vi "FW shifter.vi"() -> (0 "Cluster":T1)   [LabVIEW 2010, in "lib1299.lvlib"]
doc: "This is the constant for the variables used in the shift register of the firmware loader VI."
uses:
  lib1299.lvlib
  Controls/FW State.ctl
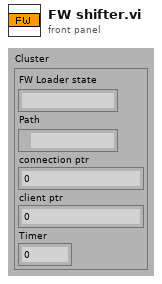
[diagram p1: front panel]
types:
  T1 = typedef "lib1299.lvlib/FW State.ctl" = cluster{"FW Loader state":string, "Path":path, "connection ptr":i32, "client ptr":i32, "Timer":i64}
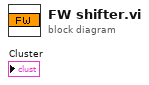
[diagram p0: block diagram]
diagram:
